vi "Initialize.vi"(4 "Y通道":string, 6 "X通道":string, 7 "原始采样率[Hz]":i32, 8 "error in (no error)":errorcluster caption="错误输入（无错误）", 9 "引用":T1, 10 "显示采样率[Hz]":i32, 11 "XYPlot 输入":refnum<class "XYPlot.lvclass">) -> (0 "error out":errorcluster caption="错误输出", 3 "XYPlot 输出":refnum<class "XYPlot.lvclass">)   [LabVIEW 2018, in "DataDisplay.lvlib" / "XYPlot.lvclass"]
uses:
  XYPlot.lvclass
  XYPlotRef.ctl
  TypeDefine/DD_DataStream.ctl
  <vilib>/Utility/miscctls.llb/LVPointTypeDef.ctl
  TypeDefine/DD_Command.ctl
  XYPlot.lvclass/XYPlot.ctl
  SubVI/DD_Parameter.vi
  DataDisplay.lvlib
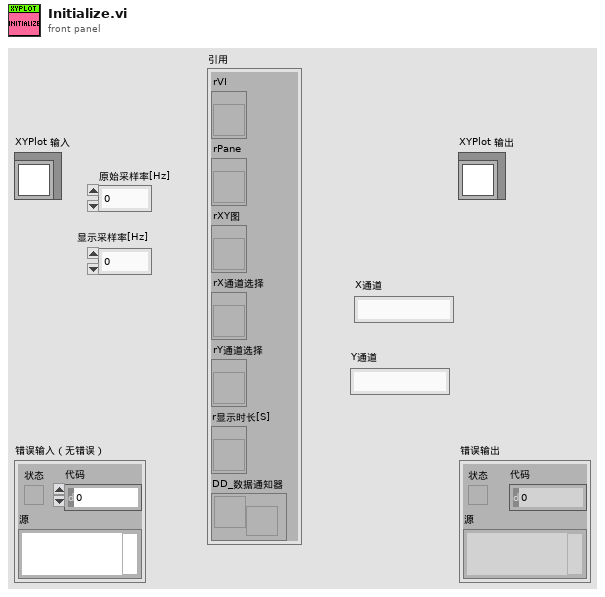
[diagram p1: front panel]
types:
  T1 = typedef "DataDisplay.lvlib/XYPlot.lvclass/XYPlotRef.ctl" = cluster{"rVI":refnum<vi>, "rPane":refnum<vi>, "rXY图":refnum<vi>, "rX通道选择":refnum<vi>, "rY通道选择":refnum<vi>, "r显示时长[S]":refnum<vi>, "DD_数据通知器":refnum<notifier>}
  T2 = typedef "DataDisplay.lvlib/DD_Command.ctl" = cluster{"消息":string, "参数":variant}
  T3 = typedef "LVPointTypeDef.ctl" = cluster{"Horizontal":i16, "Vertical":i16}
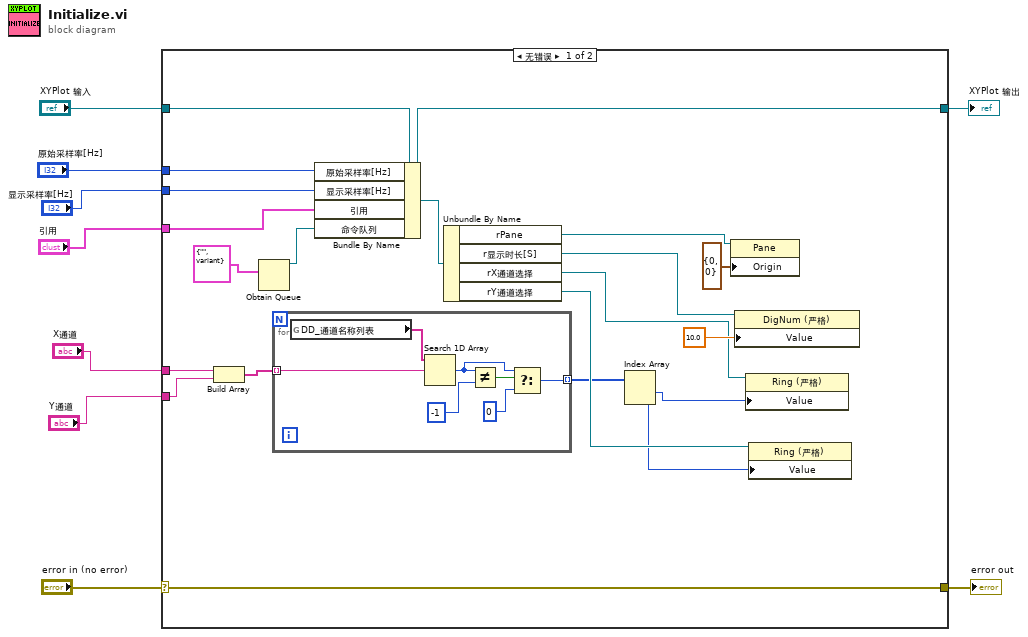
[diagram p0: block diagram]
diagram:
  n1 = case shown="无错误" "error in (no error)" {
    selector: "error in (no error)" -> [w28 w38]
    tunnel: [w28 w38] -> w8
    tunnel: [w27 w37] -> w6
    tunnel: "XYPlot 输入" -> [w29 w37]
    tunnel: "显示采样率[Hz]" -> [w26 _]
    tunnel: "引用" -> [w23 _]
    tunnel: "原始采样率[Hz]" -> [w18 _]
    tunnel: "X通道" -> [w15 _]
    tunnel: "Y通道" -> [w13 _]
    frame No Error {
      n2 = Build Array(w15, w13) -> (w14:string[])
      n3 = Obtain Queue(element data type=T2 {"消息"="", "参数"=variant} ("命令")) -> (queue out=w19:refnum<queue>)  [unwired: 4 in, 2 out]
      n4 = for {
        tunnel: [w31] -> w12 mode=indexing
        tunnel: w14 -> [w30] mode=indexing
        n5 = global read "DD_Parameter.vi" "DD_通道名称列表"() -> (w36:string[])
        n6 = Search 1D Array(1D array=w36, element=w30) -> (index of element=w33:i32)  [unwired: 1 in]
        n7 = Not Equal?(x=w33, y=-1) -> (x != y?=w34:bool)
        n8 = Select(t=w33, s=w34, f=0) -> (s? t:f=w31:i32)
      }
      n9 = Bundle By Name(cluster=w29, "原始采样率[Hz]"=w18, "显示采样率[Hz]"=w26, "引用"=w23, "命令队列"=w19) -> (w27:refnum<class "XYPlot.lvclass">)
      n10 = Unbundle By Name(w27) -> ("rPane"=w25:refnum<vi>, "r显示时长[S]"=w21:refnum<vi>, "rX通道选择"=w17:refnum<vi>, "rY通道选择"=w16:refnum<vi>)
      n11 = Index Array(array=w12) -> (element #1=w11:i32, element #2=w10:i32)  [unwired: 2 in]
      n12 = property class="Pane"(reference=w25, "Origin"=T3 {"Horizontal"=0, "Vertical"=0} ("原点")) -> ()  [unwired: 1 in, 2 out]
      n13 = property class="DigNum (严格)"(reference=w21, "Value"=10.0 ("值")) -> ()  [unwired: 1 in, 2 out]
      n14 = property class="Ring (严格)"(reference=w17, "Value"=w11) -> ()  [unwired: 1 in, 2 out]
      n15 = property class="Ring (严格)"(reference=w16, "Value"=w10) -> ()  [unwired: 1 in, 2 out]
    }
    frame Error {
    }
  }
  "error out" <- w8
  "XYPlot 输出" <- w6
